vi "Untitled 1.vi"() -> ()   [LabVIEW 2024]
panel:
  out "subarray":i32[](array[numeric])
  out "x*y":i8
  out "Numeric 2":i32
  out "x-y":dbl
  out "Numeric":i32
  out "x > y?":bool
  out "x+1":i32
  out "Array":i32[](array[numeric])
  out "deleted portion":i32
  out "array w/ subset deleted":i32[](array[numeric])
  # "1."
  # "3."
  # "4."
  # "8."
  # "12."
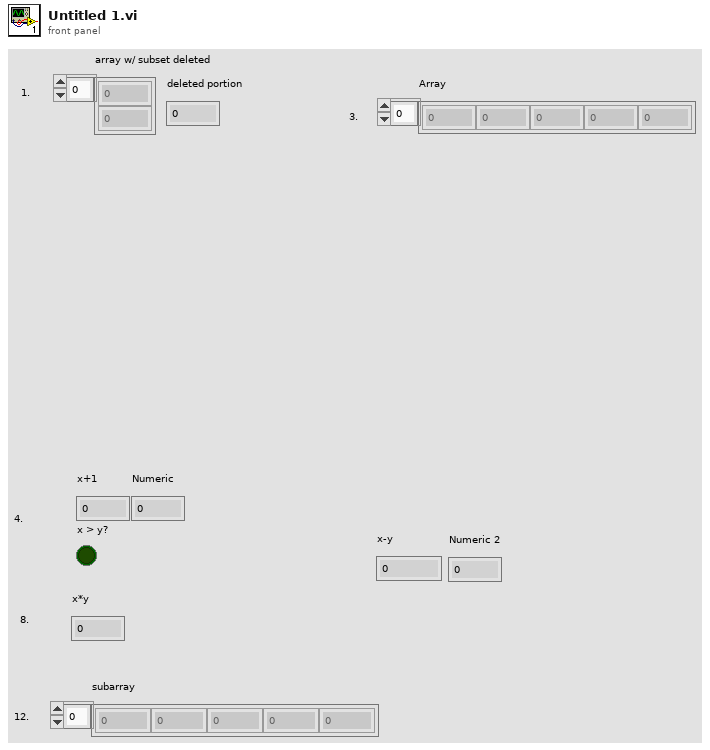
[diagram p1: front panel]
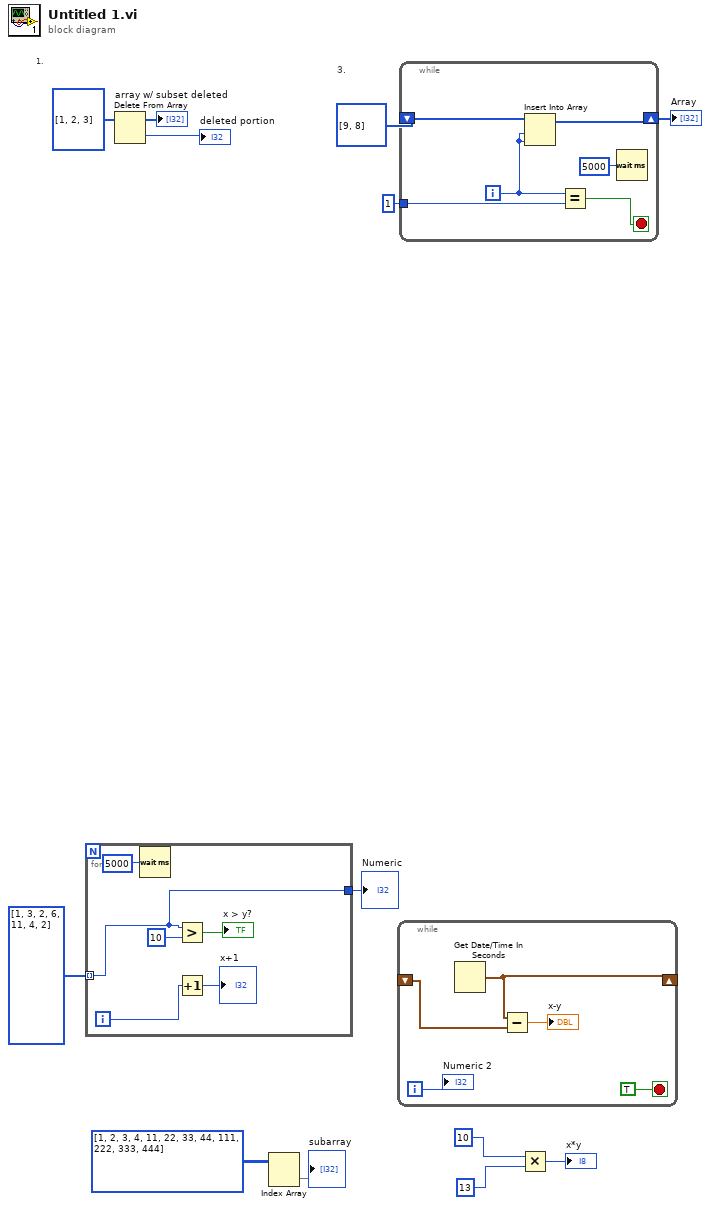
[diagram p0: block diagram]
diagram:
  # "3."
  # "1."
  n1 = for {
    tunnel: i32[] [1, 3, 2, 6, 11, 4, 2] -> [w15] mode=indexing
    tunnel: [w15] -> w9
    i -> [w19]
    n2 = Wait (ms)(milliseconds to wait=u32 5000 ("millisecond timer value")) -> ()  [unwired: 1 out]
    n3 = Greater?(x=w15, y=10) -> (0:→"x > y?":bool)
    n4 = Increment(x=w19) -> (x+1=→"x+1":i32)
  }
  "Numeric" <- w9
  n5 = Delete From Array(array=i32[] [1, 2, 3]) -> (deleted portion=→"deleted portion":i32, array with subset deleted=→"array w/ subset deleted":i32[])  [unwired: 2 in]
  n6 = Index Array(array=i32[][] [[1, 2, 3, 4], [11, 22, 33, 44], [111, 222, 333, 444]]) -> (element=→"subarray":i32[])  [unwired: 2 in]
  n7 = while {
    shift-right: [w23] -> _
    shift-left: _ -> [w24]
    i -> [w21]
    stop <- TRUE stop-if-true
    n8 = Get Date/Time In Seconds() -> (seconds since 1Jan1904=w23:timestamp)
    n9 = Subtract(x=w23, y=w24) -> (x-y=→"x-y":dbl)
    "Numeric 2" <- w21
  }
  n10 = while {
    shift-right: [w29] -> w12
    shift-left: i32[] [9, 8] -> [w25]
    tunnel: 1 -> [w27]
    i -> [w28]
    stop <- w30 stop-if-true
    n11 = Insert Into Array(array=w25, index=w28, new element=w28) -> (w29:i32[])
    n12 = Equal?(x=w28, y=w27) -> (x = y?=w30:bool)
    n13 = Wait (ms)(milliseconds to wait=u32 5000 ("millisecond timer value")) -> ()  [unwired: 1 out]
  }
  "Array" <- w12
  n14 = Multiply(x=10, y=13) -> (x*y=→"x*y":i32)
